vi "JSON No Whitespace.vi"(0 "String":string, 1 "Except in Quotes (F)":bool) -> (2 "Trimmed String":string)   [LabVIEW 2013, in "LV JSON.lvlib"]
doc: "Remove all whitespace from String. To keep whitespace inside of quotation marks set Except in Quotes (F) to True."
uses:
  LV JSON.lvlib
panel:
  out "String 2":string
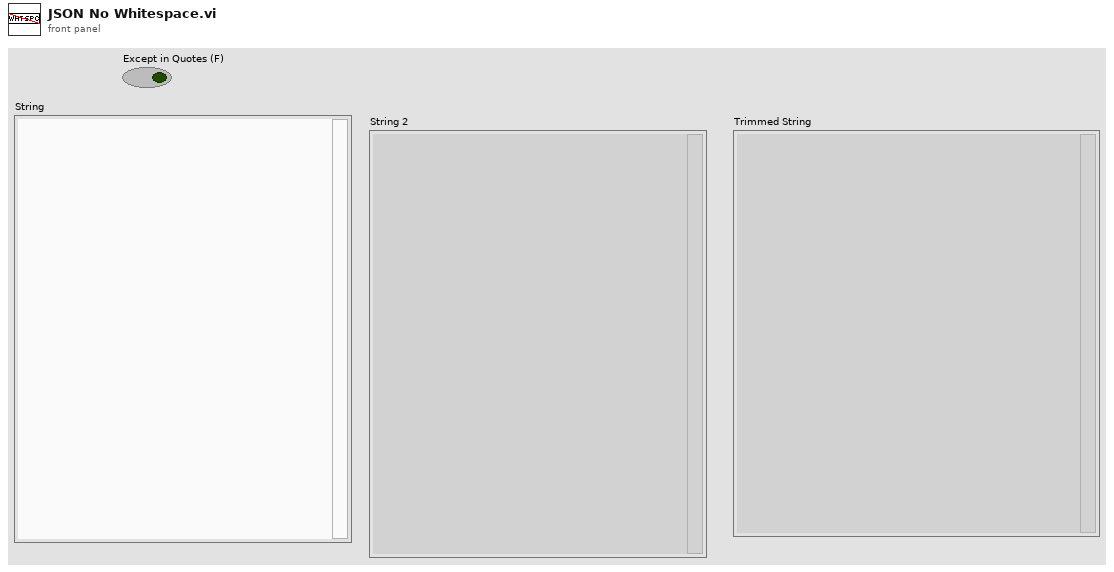
[diagram p1: front panel]
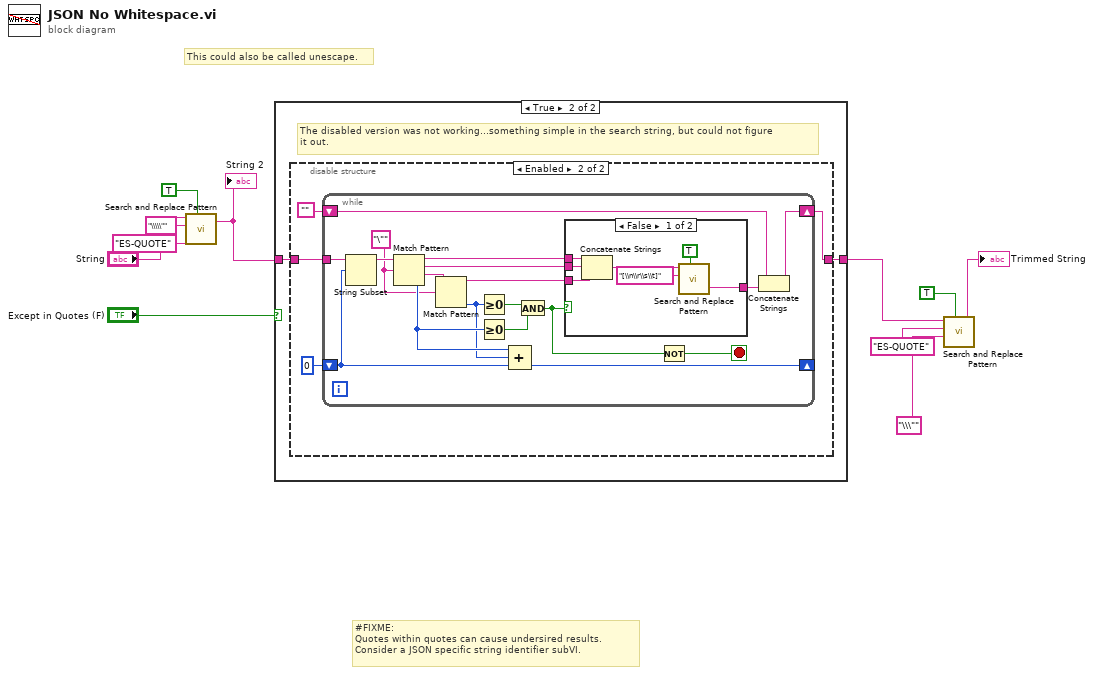
[diagram p0: block diagram]
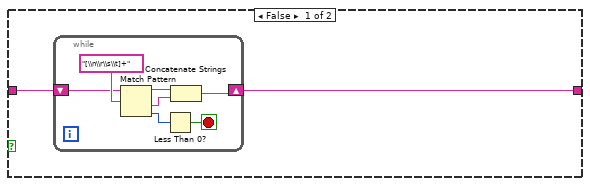
[diagram p2: hidden frame]
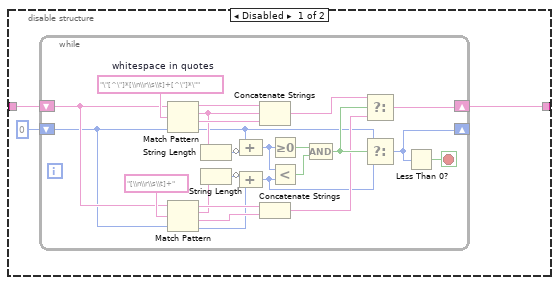
[diagram p3: hidden frame]
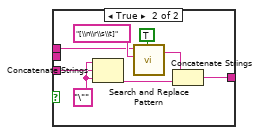
[diagram p4: hidden frame]
diagram:
  # "This could also be called unescape."
  # "#FIXME:\nQuotes within quotes can cause undersired results.\nConsider a JSON specific string identifier subVI."
  n1 = call <vilib>:"Search and Replace Pattern.vi"("string"="String", "regular expression (\"\")"="\\\\\"" ("regular expression (\"\")"), "replace string (\"\")"="ES-QUOTE" ("replace string (\"\")"), "replace all? (F)"=TRUE) -> ("result string"=w2:string)  [unwired: 1 in, 1 out]
  "String 2" <- w2
  n2 = case shown="True" "Except in Quotes (F)" {
    tunnel: [w12 w22] -> w4
    tunnel: w2 -> [w13 w21]
    frame False {
      n3 = while {
        shift-right: [w15] -> w12
        shift-left: w13 -> [w18]
        stop <- w20 stop-if-true
        n4 = Match Pattern(string=w18, regular expression="[\\n\\r\\s\\t]+") -> (before substring=w17:string, after substring=w16:string, offset past match=w14:i32)  [unwired: 1 in, 1 out]
        n5 = Less Than 0?(x=w14) -> (x < 0?=w20:bool)
        n6 = Concatenate Strings(w17, w16) -> (w15:string)
      }
    }
    frame True {
      # "The disabled version was not working...something simple in the search string, but could not figure\nit out."
      n7 = disable-structure shown="Enabled" {
        disable-tunnel: [w25 w52] -> w22
        disable-tunnel: w21 -> [w23 w53]
        frame Disabled {
          n8 = while {
            shift-right: [w37] -> w25
            shift-left: w23 -> [w44]
            shift-right: [w36] -> _
            shift-left: 0 ("offset past match") -> [w43]
            stop <- w47 stop-if-true
            w49 = "\"[^\"]*[\\n\\r\\s\\t]+[^\"]*\""  # whitespace in quotes
            n9 = Match Pattern(string=w44, regular expression=w49, offset (0)=w43) -> (before substring=w48:string, match substring=w35:string, after substring=w46:string, offset past match=w32:i32)
            n10 = Match Pattern(string=w44, regular expression="[\\n\\r\\s\\t]+", offset (0)=w43) -> (before substring=w30:string, match substring=w29:string, after substring=w39:string, offset past match=w27:i32)
            n11 = String Length(string=w35) -> (length=w33:i32)
            n12 = String Length(string=w29) -> (length=w28:i32)
            n13 = Compound Arithmetic op=ADD(w32, invert w33) -> (w31:i32)
            n14 = Compound Arithmetic op=ADD(invert w28, w27) -> (w26:i32)
            n15 = Concatenate Strings(w48, w35, w46) -> (w40:string)
            n16 = Concatenate Strings(w30, w39) -> (w38:string)
            n17 = Greater Or Equal To 0?(x=w31) -> (x >= 0?=w34:bool)
            n18 = Less?(x=w31, y=w26) -> (x < y?=w42:bool)
            n19 = Compound Arithmetic op=AND(w34, w42) -> (w41:bool)
            n20 = Select(t=w40, s=w41, f=w38) -> (s? t:f=w37:string)
            n21 = Select(t=w32, s=w41, f=w26) -> (s? t:f=w36:i32)
            n22 = Less Than 0?(x=w36) -> (x < 0?=w47:bool)
          }
        }
        frame Enabled {
          n23 = while {
            tunnel: w53 -> [w71]
            shift-right: [w60] -> w52
            shift-left: "" -> [w61]
            shift-right: [w54] -> _
            shift-left: 0 -> [w55]
            stop <- w63 stop-if-true
            w56 = "\"" ("string")
            n24 = String Subset(string=w71, offset (0)=w55) -> (substring=w59:string)  [unwired: 1 in]
            n25 = Match Pattern(string=w59, regular expression=w56) -> (before substring=w67:string, match substring=w65:string, after substring=w70:string, offset past match=w58:i32)  [unwired: 1 in]
            n26 = Match Pattern(string=w70, regular expression=w56) -> (before substring=w66:string, offset past match=w57:i32)  [unwired: 1 in, 2 out]
            n27 = Greater Or Equal To 0?(x=w57) -> (x >= 0?=w69:bool)
            n28 = Greater Or Equal To 0?(x=w58) -> (x >= 0?=w68:bool)
            n29 = Compound Arithmetic op=ADD(w58, w57, w55) -> (w54:i32)
            n30 = And(x=w69, y=w68) -> (x .and. y?=w64:bool)
            n31 = case shown="False" w64 {
              tunnel: w67 -> [w78 w85]
              tunnel: w66 -> [w76 w82]
              tunnel: [w72 w79] -> w62
              tunnel: w65 -> [w77 _]
              frame False {
                n32 = Concatenate Strings(w78, w77, w76) -> (w73:string)
                n33 = call <vilib>:"Search and Replace Pattern.vi"("string"=w73, "regular expression (\"\")"="[\\n\\r\\s\\t]" ("regular expression (\"\")"), "replace all? (F)"=TRUE) -> ("result string"=w72:string)  [unwired: 2 in, 1 out]
              }
              frame True {
                w83 = "\"" ("string")
                n34 = Concatenate Strings(w83, w82, w83) -> (w80:string)
                n35 = call <vilib>:"Search and Replace Pattern.vi"("string"=w85, "regular expression (\"\")"="[\\n\\r\\s\\t]" ("regular expression (\"\")"), "replace all? (F)"=TRUE) -> ("result string"=w81:string)  [unwired: 2 in, 1 out]
                n36 = Concatenate Strings(w81, w80) -> (w79:string)
              }
            }
            n37 = Not(x=w64) -> (.not. x?=w63:bool)
            n38 = Concatenate Strings(w61, w62) -> (w60:string)
          }
        }
      }
    }
  }
  n39 = call <vilib>:"Search and Replace Pattern.vi"("string"=w4, "regular expression (\"\")"="ES-QUOTE" ("replace string (\"\")"), "replace string (\"\")"="\\\"" ("regular expression (\"\")"), "replace all? (F)"=TRUE) -> ("result string"=→"Trimmed String":string)  [unwired: 1 in, 1 out]
